vi "Climbing.vi"(8 "Joystick In":dbl) -> (0 "Override":bool, 1 "Climb Speed":dbl)   [LabVIEW 2016]
uses:
  Robot Global Data.vi
  <vilib>/Rock Robotics/Network Tables/NT Write Boolean.vi
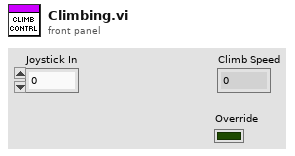
[diagram p1: front panel]
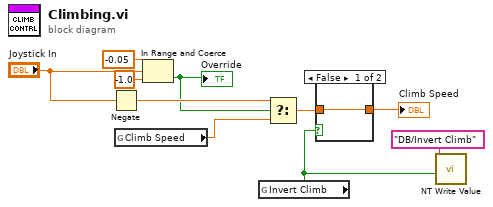
[diagram p0: block diagram]
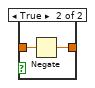
[diagram p2: hidden frame]
diagram:
  n1 = Negate(x="Joystick In") -> (-x=w5:dbl)
  n2 = global read "Robot Global Data.vi" "Climb Speed"() -> (w9:dbl)
  n3 = In Range and Coerce(upper limit=-0.05, x="Joystick In", lower limit=-1.0) -> (In Range?=w4:bool)  [unwired: 1 out]
  "Override" <- w4
  n4 = global read "Robot Global Data.vi" "Invert Climb"() -> (w1:bool)
  n5 = Select(t=w5, s=w4, f=w9) -> (s? t:f=w10:dbl)
  n6 = case shown="False" w1 {
    tunnel: w10 -> [w11 w13]
    tunnel: [w11 w12] -> w3
    frame False {
    }
    frame True {
      n7 = Negate(x=w13) -> (-x=w12:dbl)
    }
  }
  "Climb Speed" <- w3
  n8 = call-poly <vilib>:"NT Write Value.vi"("Boolean"=w1, "Name"="DB/Invert Climb") -> ()  [unwired: 9 in, 1 out]
